vi "Intake_Var.vi"(1 "DIO":T1) -> (0 "Intake Var":T10)   [LabVIEW 2015]
uses:
  Ref_Num/DIO_Type_Def.ctl
  <vilib>/Rock Robotics/WPI/Ultrasonic/WPI_SonarMB1010DigitalDeviceRef.ctl
  <vilib>/Rock Robotics/WPI/Counter/WPI_CounterDevRef.ctl
  <vilib>/Rock Robotics/SystemInterfaces/Counter/FPGA_CounterCtrSystemIndex.ctl
  <vilib>/Rock Robotics/WPI/Encoder/WPI_EncoderDevRef.ctl
  <vilib>/Rock Robotics/SystemInterfaces/Encoder/FPGA_EncoderIdx.ctl
  <vilib>/Rock Robotics/WPI/Encoder/WPI_EncoderType.ctl
  <vilib>/Rock Robotics/WPI/DigitalInput/WPI_DigitalInputDevRef.ctl
  <vilib>/Rock Robotics/SystemInterfaces/DIO/FPGA_DIOChannel.ctl
  Global_Var/JoyStick_Global.vi
panel:
  # "Created by Matt Carr\non 8 Febuary 2016"
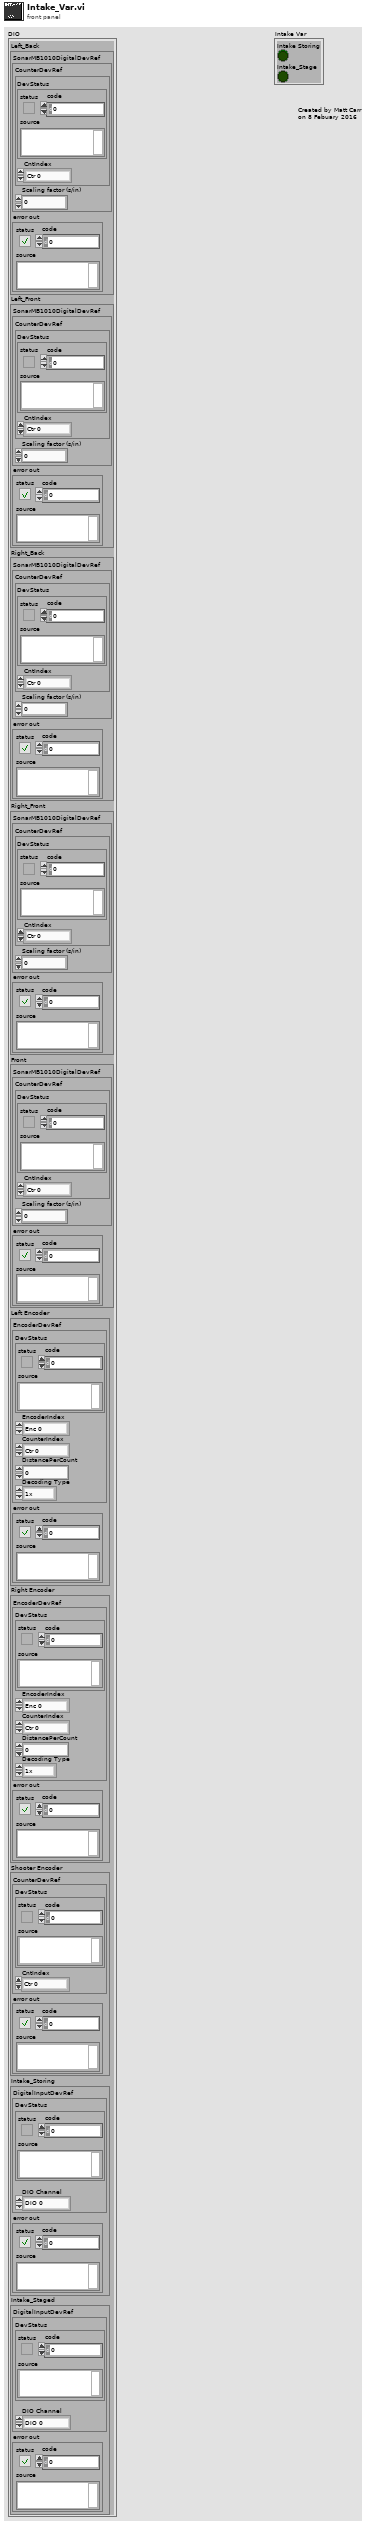
[diagram p1: front panel]
types:
  T1 = typedef "DIO_Type_Def.ctl" = cluster{"Left_Back":cluster{"SonarMB1010DigitalDevRef":T2, "error out":errorcluster}, "Left_Front":cluster{"SonarMB1010DigitalDevRef":T2, "error out":errorcluster}, "Right_Back":cluster{"SonarMB1010DigitalDevRef":T2, "error out":errorcluster}, "Right_Front":cluster{"SonarMB1010DigitalDevRef":T2, "error out":errorcluster}, "Front":cluster{"SonarMB1010DigitalDevRef":T2, "error out":errorcluster}, "Left Encoder":cluster{"EncoderDevRef":T5, "error out":errorcluster}, "Right Encoder":cluster{"EncoderDevRef":T5, "error out":errorcluster}, "Shooter Encoder":cluster{"CounterDevRef":T3, "error out":errorcluster}, "Intake_Storing":cluster{"DigitalInputDevRef":T8, "error out":errorcluster}, "Intake_Staged":cluster{"DigitalInputDevRef":T8, "error out":errorcluster}}
  T2 = typedef "WPI_SonarMB1010DigitalDeviceRef.ctl" = cluster{"CounterDevRef":T3, "Scaling factor (s/in)":dbl}
  T3 = typedef "WPI_CounterDevRef.ctl" = cluster{"DevStatus":errorcluster, "CntIndex":T4}
  T4 = typedef "FPGA_CounterCtrSystemIndex.ctl" = enum8{"Ctr 0", "Ctr 1", "Ctr 2", "Ctr 3", "Ctr 4", "Ctr 5", "Ctr 6", "Ctr 7", "Invalid"}
  T5 = typedef "WPI_EncoderDevRef.ctl" = cluster{"DevStatus":errorcluster, "EncoderIndex":T6, "CounterIndex":T4, "DistancePerCount":dbl, "Decoding Type":T7}
  T6 = typedef "FPGA_EncoderIdx.ctl" = enum8{"Enc 0", "Enc 1", "Enc 2", "Enc 3", "Enc 4", "Enc 5", "Enc 6", "Enc 7", "Invalid"}
  T7 = typedef "WPI_EncoderType.ctl" = enum16{"1x", "2x", "4x"}
  T8 = typedef "WPI_DigitalInputDevRef.ctl" = cluster{"DevStatus":errorcluster, "DIO Channel":T9}
  T9 = typedef "FPGA_DIOChannel.ctl" = enum8{"DIO 0", "DIO 1", "DIO 2", "DIO 3", "DIO 4", "DIO 5", "DIO 6", "DIO 7", "DIO 8", "DIO 9", "DIO MXP 0", "DIO MXP 1", "DIO MXP 2", "DIO MXP 3", "DIO MXP 4", "DIO MXP 5", "DIO MXP 6", "DIO MXP 7", "DIO MXP 8", "DIO MXP 9", "DIO MXP 10", "DIO MXP 11", "DIO MXP 12", "DIO MXP 13", "DIO MXP 14", "DIO MXP 15", "Invalid"}
  T10 = cluster{"Intake Storing":bool, "Intake_Stage":bool}
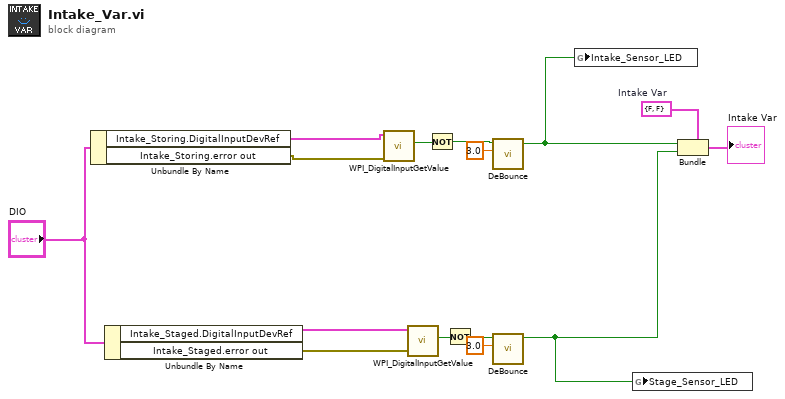
[diagram p0: block diagram]
diagram:
  w11 = T10 {"Intake Storing"=FALSE, "Intake_Stage"=FALSE}  # Intake Var
  n1 = Unbundle By Name("DIO") -> ("Intake_Storing.DigitalInputDevRef"=w15:T8, "Intake_Storing.error out"=w14:errorcluster)
  n2 = Unbundle By Name("DIO") -> ("Intake_Staged.DigitalInputDevRef"=w13:T8, "Intake_Staged.error out"=w12:errorcluster)
  n3 = call <vilib>:"WPI_DigitalInputGetValue.vi"("error in (no error)"=w14, "DigitalInputDevRef"=w15) -> ("Value"=w7:bool)  [unwired: 7 in, 2 out]
  n4 = call <vilib>:"WPI_DigitalInputGetValue.vi"("error in (no error)"=w12, "DigitalInputDevRef"=w13) -> ("Value"=w5:bool)  [unwired: 7 in, 2 out]
  n5 = Not(x=w7) -> (.not. x?=w6:bool)
  n6 = Not(x=w5) -> (.not. x?=w4:bool)
  n7 = call "DeBounce.vi"("DB_Count"=3.0, "Value"=w6) -> ("BD_Value"=w2:bool)  [unwired: 9 in]
  n8 = call "DeBounce.vi"("DB_Count"=3.0, "Value"=w4) -> ("BD_Value"=w1:bool)  [unwired: 9 in]
  n9 = global write "JoyStick_Global.vi" "Intake_Sensor_LED"(w2) -> ()
  n10 = global write "JoyStick_Global.vi" "Stage_Sensor_LED"(w1) -> ()
  n11 = Bundle(cluster=w11, "Intake Storing"=w2, "Intake_Stage"=w1) -> (→"Intake Var":T10)
